vi "set Stats.vi"(10 "Stats":T1 {"Delta Time" format="%.0p"; "Frame Rate" format="%.0p"; "Present Duration" format="%.0p"; "Raster Duration" format="%.0p"; "Transform And Project Duration" format="%.0p"}, 11 "Scene in":refnum<class "Scene.lvclass">) -> (3 "Scene out":refnum<class "Scene.lvclass">)   [LabVIEW 2020, in "Scene.lvclass"]
uses:
  Scene.lvclass
  Scene.lvclass/Scene.ctl
  Stats.ctl
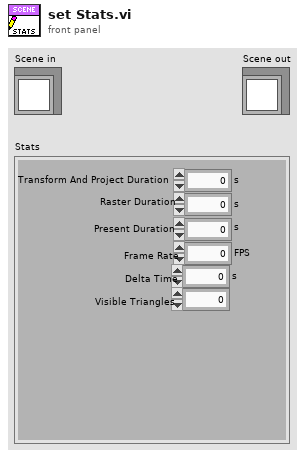
[diagram p1: front panel]
types:
  T1 = typedef "Scene.lvclass/Stats.ctl" = cluster{"Transform And Project Duration":dbl, "Raster Duration":dbl, "Present Duration":dbl, "Frame Rate":dbl, "Visible Triangles":i32, "Delta Time":dbl}
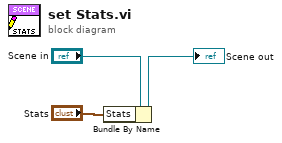
[diagram p0: block diagram]
diagram:
  n1 = Bundle By Name(cluster="Scene in", "Stats"="Stats") -> (→"Scene out":refnum<class "Scene.lvclass">)
